vi "8.5-Test of Comm Protocol.vi"() -> ()   [LabVIEW 2010]
uses:
  2-Low Neurons/2.2-Where Control.ctl
  2-Low Neurons/2.2-Where Indicator.ctl
panel:
  in  "End Graph":bool
  out "Waveform Chart":cluster{"New Local Clock: Clk":i8, "Clk":i8}(graph)
  out "RT State":enum16{"Send", "Receive"}(ring)
  out "unsigned byte array":u8[](array[numeric])
  out "Data Byte to Send":u8
  out "Data going to serial":u8
  out "Left to write":i32
  in  "ICs for RT":T1
  out "Send New Data":bool
  out "Store New Data":bool
  out "Out of Message":bool
  in  "Begin RT":bool
  out "RT Clk Mem":i8
  out "RS232-1\\Port1 Write Case":bool
  out "Observed Reply":string
  in  "Prepared Command to Device":string
  in  "stop \"RT Target\"":bool
  out "Observed Command on Device":u8[](array[numeric])
  in  "Prepared Reply on Device":u8[](array[numeric])=[0, 0, 0, 0]
  in  "stop \"FPGA\"":bool
  out "2.2 Where Indicator":T2
  in  "2.2 Where Control":T1
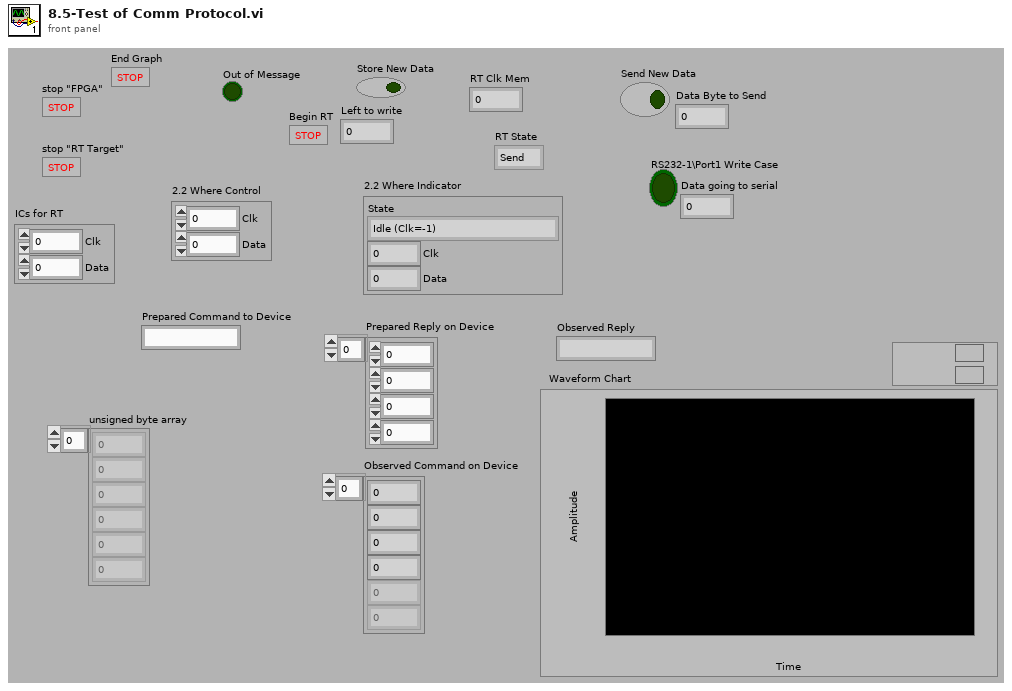
[diagram p1: front panel]
types:
  T1 = typedef "2.2-Where Control.ctl" = cluster{"Clk":i8, "Data":u8}
  T2 = typedef "2.2-Where Indicator.ctl" = cluster{"State":enum8{"Idle (Clk=-1)", "Sending(Clk*==Clk+1?Clk=Clk*:;)", "Receiving(Clk*==Clk?Clk++:;)"}, "Clk":i8, "Data":u8}
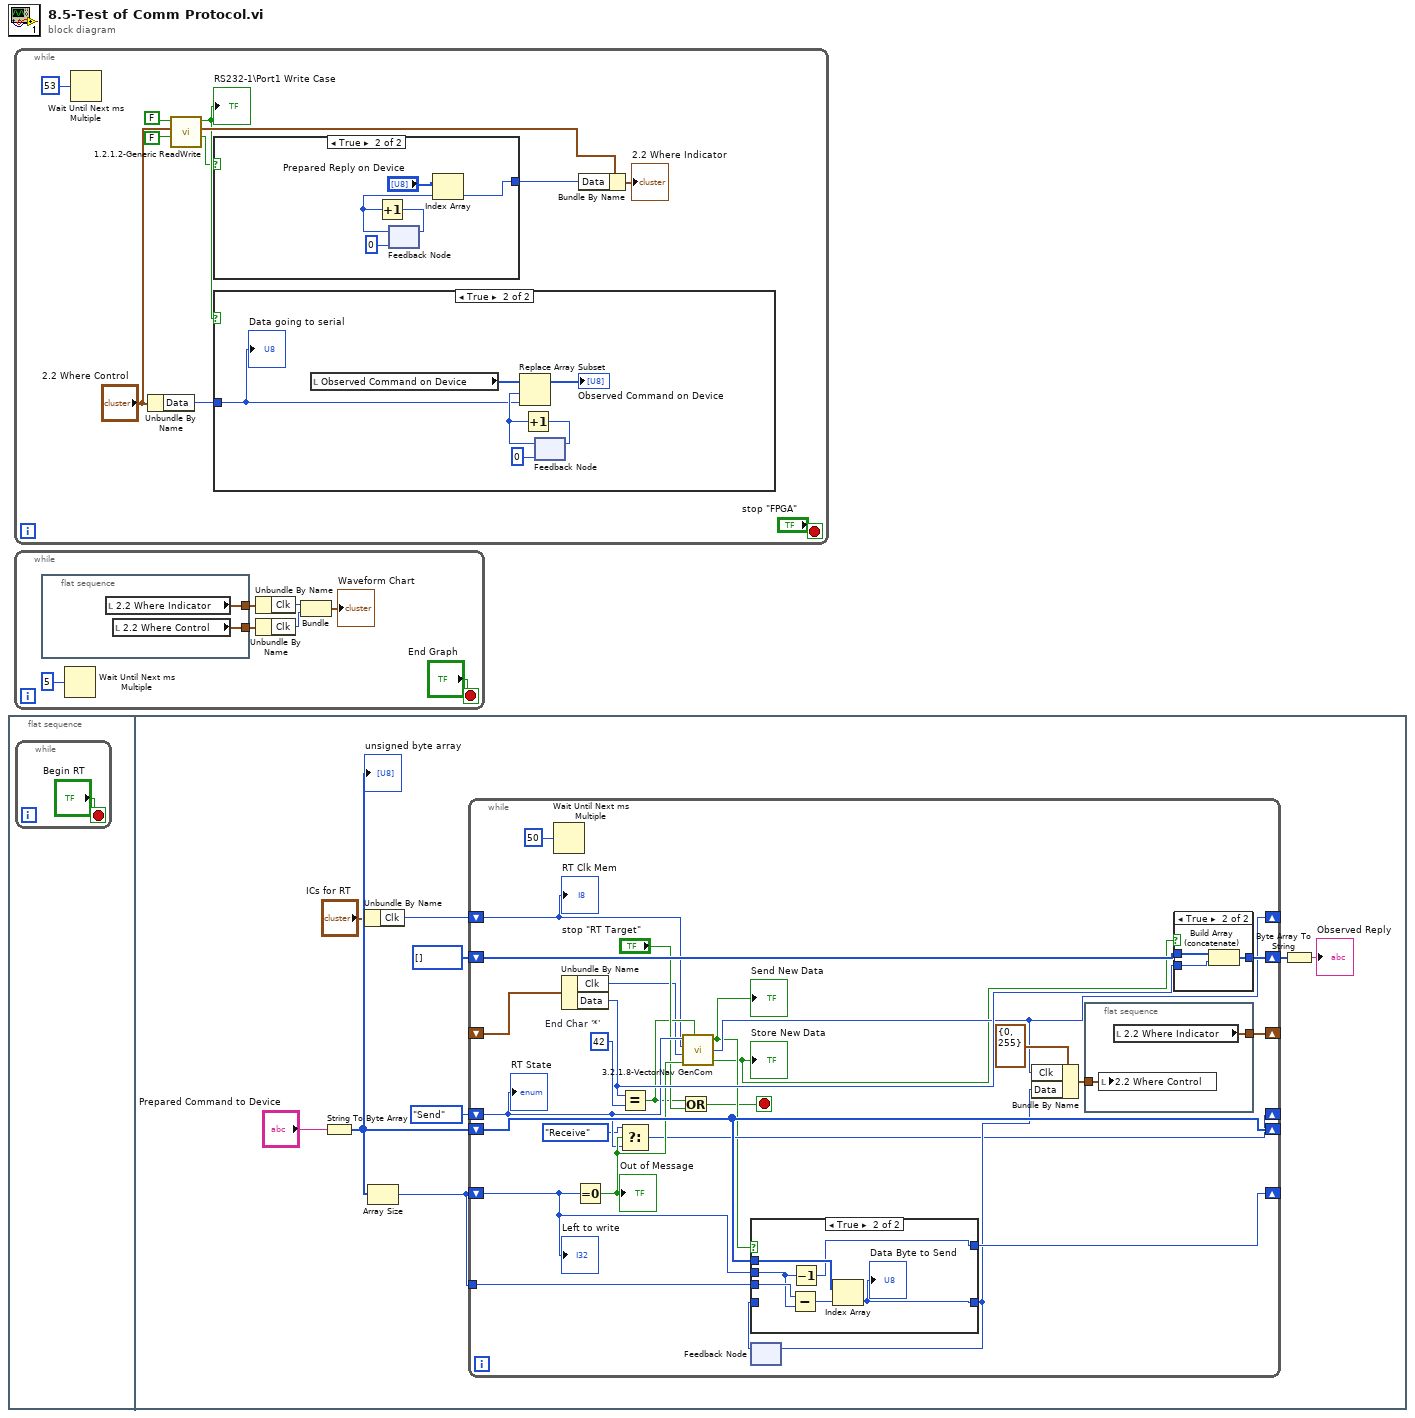
[diagram p0: block diagram]
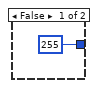
[diagram p4: hidden frame]
diagram:
  n1 = flat-sequence {
    frame #0 {
      n2 = while {
        stop <- "Begin RT" stop-if-true
      }
    }
    frame #1 {
      n3 = String To Byte Array(string="Prepared Command to Device") -> (unsigned byte array=w7:u8[])
      "unsigned byte array" <- w7
      n4 = Unbundle By Name("ICs for RT") -> ("Clk"=w4:i8)
      n5 = Array Size(array=w7) -> (size(s)=w3:i32)
      n6 = while {
        shift-right: [w35] -> _
        shift-left: w7 -> [w35]
        shift-right: [w33] -> w2
        shift-left: u8[] [] ("unsigned byte array") -> [w34]
        shift-right: [w31] -> _
        shift-left: w3 -> [w28]
        shift-right: [w26] -> _
        shift-left: _ -> [w27]
        shift-right: [w24] -> _
        shift-left: w4 -> [w12]
        shift-right: [w20] -> _
        shift-left: enum16{"Send", "Receive"}."Send" ("State") -> [w22]
        tunnel: w3 -> [w18]
        stop <- w14 stop-if-true
        w25 = u8 42  # End Char '*'
        n7 = Wait Until Next ms Multiple(millisecond multiple=u32 50) -> ()  [unwired: 1 out]
        n8 = Unbundle By Name(w27) -> ("Clk"=w11:i8, "Data"=w32:u8)
        n9 = Equal To 0?(x=w28) -> (x = 0?=w23:bool)
        "Out of Message" <- w23
        n10 = Equal?(x=w32, y=w25) -> (x = y?=w13:bool)
        n11 = Select(t=enum16{"Send", "Receive"}."Receive", s=w23, f=w22) -> (s? t:f=w20:enum16{"Send", "Receive"})
        n12 = Or(x=w13, y="stop \"RT Target\"") -> (x .or. y?=w14:bool)
        n13 = call "3.2.1.8-VectorNav GenCom.vi"("State"=w22, "Local Clock: Clk"=w12, "Foreign Clock: Clk*"=w11, "Out of Message"=w23, "This is the Last Byte to Read"=w13) -> ("Send New Data"=w17:bool, "New Local Clock: Clk"=w24:i8, "Store New Data"=w16:bool)
        "Store New Data" <- w16
        "Send New Data" <- w17
        n14 = feedback #1() -> (w29:u8)  [unwired: 1 in]
        n15 = case shown="True" w17 {
          tunnel: w35 -> [_ w51]
          tunnel: [w44 w50] -> w30
          tunnel: [w45 w47] -> w31
          tunnel: w28 -> [w45 w46]
          tunnel: w29 -> [w44 _]
          tunnel: w18 -> [_ w49]
          frame False {
          }
          frame True {
            n16 = Subtract(x=w49, y=w46) -> (x-y=w48:i32)
            n17 = Decrement(x=w46) -> (x-1=w47:i32)
            n18 = Index Array(array=w51, index=w48) -> (element=w50:u8)
            "Data Byte to Send" <- w50
          }
        }
        n19 = feedback-in #1(w30) -> ()
        n20 = Bundle By Name(cluster=T1 {"Clk"=0, "Data"=255} ("2.2 Where Control"), "Clk"=w24, "Data"=w30) -> (w36:T1)
        n21 = flat-sequence "FPGA Interface" {
          tunnel: w36 -> [w38]
          tunnel: [w39] -> w26
          frame #0 {
            n22 = local write "2.2 Where Control"(w38) -> ()
            n23 = local read "2.2 Where Indicator"() -> (w39:T2)
          }
        }
        n24 = case shown="True" w16 {
          tunnel: w34 -> [w40 w43]
          tunnel: [w40 w42] -> w33
          tunnel: w32 -> [_ w41]
          frame False {
          }
          frame True {
            n25 = Build Array (concatenate)(w43, w41) -> (w42:u8[])
          }
        }
        "RT Clk Mem" <- w12
        "Left to write" <- w28
        "RT State" <- w22
      }
      n26 = Byte Array To String(unsigned byte array=w2) -> (string=→"Observed Reply":string)
    }
  }
  n27 = while {
    stop <- "stop \"FPGA\"" stop-if-true
    n28 = Wait Until Next ms Multiple(millisecond multiple=u32 53) -> ()  [unwired: 1 out]
    n29 = Unbundle By Name("2.2 Where Control") -> ("Data"=w54:u8)
    n30 = call "1.2.1.2-Generic ReadWrite.vi"("RS232-1\\Port1 Read Timeout"=FALSE ("RS232-1\\Port1 Read Timeout"), "2.2 Where Control"="2.2 Where Control", "RS232-1\\Port1 Write Timeout"=FALSE ("RS232-1\\Port1 Write Timeout")) -> ("RS232-1\\Port1 Read Case"=w57:bool, "2.2 Where Indicator"=w61:T2, "RS232-1\\Port1 Write Case"=w58:bool)  [unwired: 2 in]
    "RS232-1\\Port1 Write Case" <- w58
    n31 = case shown="True" w57 {
      tunnel: [u8 255 ("Numeric") w64] -> w56
      frame False {
      }
      frame True {
        n32 = feedback #2(0) -> (w67:i32)
        n33 = Increment(x=w67) -> (x+1=w66:i32)
        n34 = feedback-in #2(w66) -> ()
        n35 = Index Array(array="Prepared Reply on Device", index=w67) -> (element=w64:u8)
      }
    }
    n36 = case shown="True" w58 {
      tunnel: w54 -> [_ w69]
      frame False {
      }
      frame True {
        n37 = local read "Observed Command on Device"() -> (w74:u8[])
        n38 = feedback #3(0) -> (w70:i32)
        n39 = Replace Array Subset(array=w74, new element=w69, index=w70) -> (→"Observed Command on Device":u8[])
        n40 = Increment(x=w70) -> (x+1=w71:i32)
        n41 = feedback-in #3(w71) -> ()
        "Data going to serial" <- w69
      }
    }
    n42 = Bundle By Name(cluster=w61, "Data"=w56) -> (→"2.2 Where Indicator":T2)
  }
  n43 = while {
    stop <- "End Graph" stop-if-true
    n44 = flat-sequence "FPGA Interface" {
      tunnel: [w83] -> w80
      tunnel: [w82] -> w79
      frame #0 {
        n45 = local read "2.2 Where Indicator"() -> (w83:T2)
        n46 = local read "2.2 Where Control"() -> (w82:T1)
      }
    }
    n47 = Wait Until Next ms Multiple(millisecond multiple=u32 5) -> ()  [unwired: 1 out]
    n48 = Unbundle By Name(w80) -> ("Clk"=w78:i8)
    n49 = Unbundle By Name(w79) -> ("Clk"=w77:i8)
    n50 = Bundle("Clk"=w78, "Clk"=w77) -> (→"Waveform Chart":cluster{"Clk":i8, "Clk":i8})  [unwired: 1 in]
  }
